vi "Set DAQ cards to max convert.vi"(8 "error in (no error)":errorcluster, 11 "Target":refnum<k24>) -> (0 "error out":errorcluster, 3 "Target dup":refnum<k24>)   [LabVIEW 2011]
uses:
  NationalInstruments.VeriStand.SystemDefinitionAPI
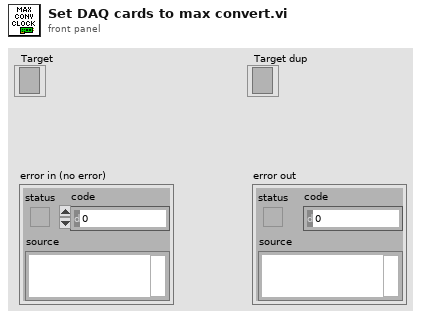
[diagram p1: front panel]
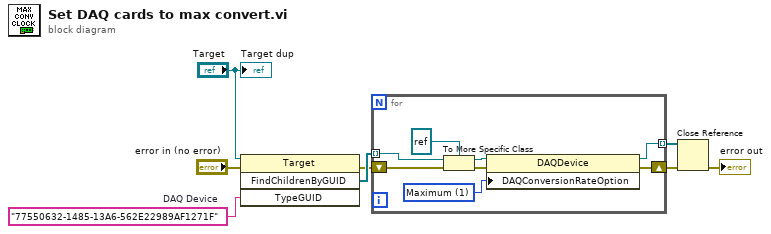
[diagram p0: block diagram]
diagram:
  w8 = "77550632-1485-13A6-562E22989AF1271F"  # DAQ Device
  n1 = invoke class="Target" method="FindChildrenByGUID"(reference="Target", error in="error in (no error)", "TypeGUID"=w8) -> (error out=w1:errorcluster, "FindChildrenByGUID"=w7:refnum<k24>[])  [unwired: 1 in, 2 out]
  n2 = for {
    tunnel: w7 -> [w15] mode=indexing
    shift-right: [w11] -> w6
    shift-left: w1 -> [w16]
    tunnel: [w10] -> w2 mode=indexing
    w9 = 1 items=["Default", "Maximum"] ("DAQConversionRateOption")
    n3 = To More Specific Class(target class=refnum<k24> refnum, reference=w15, error in=w16) -> (specific class reference=w12:refnum<k24>, error out=w13:errorcluster)
    n4 = property class="DAQDevice"(reference=w12, error in=w13, "DAQConversionRateOption"=w9) -> (reference out=w10:refnum<k24>, error out=w11:errorcluster)
  }
  n5 = Close Reference(reference=w2, error in (no error)=w6) -> (error out=→"error out":errorcluster)
  "Target dup" <- "Target"
